vi "BK Precision 178XB Setup Output.vi"() -> ()   [LabVIEW 2019]
doc: "This example VI demonstrates the basic configuration of the power supply. It can be used to configure the voltage and current limit for output, and enables the output once configured."
uses:
  BK Precision 178XB Series.lvlib
panel:
  in  "stop":bool
  in  "Output Voltage (0)":dbl min=0.0 max=18.0 format="%#.2f"
  in  "Current Limit (0)":dbl min=0.0 max=6.0 format="%#.2g"
  in  "Maximum Output Voltage (18)":dbl=8.0 min=0.0 max=72.0 format="%#.2f"
  in  "VISA resource name":refnum<visa-resource-name>
  # "Instructions:  Set the maximum output voltage desired for overvoltage protection.  Then configure the output voltage and the current limit.  To end, press the Stop button."
  # "(c) 2009 B&K PRECISION CORPORATION.  ALL RIGHTS RESERVED."
  # "V"
  # "A"
  # "V"
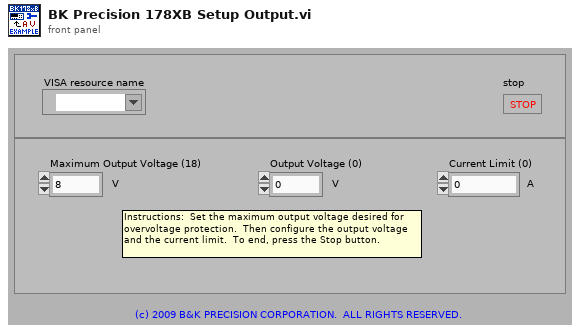
[diagram p1: front panel]
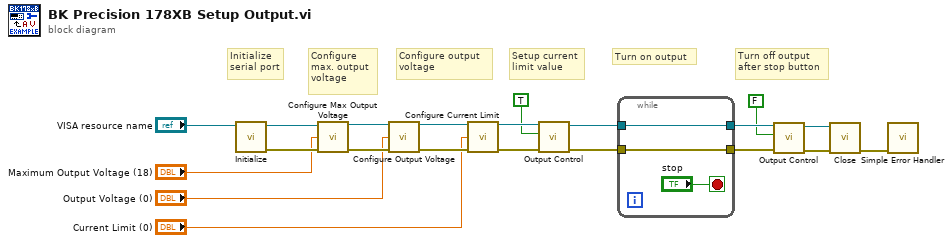
[diagram p0: block diagram]
diagram:
  # "Turn off output\nafter stop button"
  # "Turn on output"
  # "Setup current\nlimit value"
  # "Configure output\nvoltage"
  # "Configure\nmax. output\nvoltage"
  # "Initialize\nserial port"
  n1 = call "Initialize.vi"("VISA resource name"="VISA resource name") -> ("error out"=w19:errorcluster, "VISA resource name out"=w20:refnum<visa-resource-name>)  [unwired: 9 in]
  n2 = call "Configure Max Output Voltage.vi"("VISA resource name"=w20, "Maximum Output Voltage (18)"="Maximum Output Voltage (18)", "error in (no error)"=w19) -> ("VISA resource name out"=w18:refnum<visa-resource-name>, "error out"=w15:errorcluster)  [unwired: 11 in]
  n3 = call "Configure Output Voltage.vi"("VISA resource name"=w18, "Output Voltage (0)"="Output Voltage (0)", "error in (no error)"=w15) -> ("VISA resource name out"=w17:refnum<visa-resource-name>, "error out"=w16:errorcluster)  [unwired: 11 in]
  n4 = call "Configure Current Limit.vi"("VISA resource name"=w17, "Current Limit (0)"="Current Limit (0)", "error in (no error)"=w16) -> ("VISA resource name out"=w14:refnum<visa-resource-name>, "error out"=w13:errorcluster)  [unwired: 11 in]
  n5 = call "Output Control.vi"("error in (no error)"=w13, "Enable Output Terminals (F: Off)"=TRUE, "VISA resource name"=w14) -> ("error out"=w11:errorcluster, "VISA resource name out"=w12:refnum<visa-resource-name>)  [unwired: 7 in]
  n6 = while {
    tunnel: w12 -> [w24]
    tunnel: w11 -> [w23]
    tunnel: [w24] -> w5
    tunnel: [w23] -> w4
    stop <- "stop" stop-if-true
  }
  n7 = call "Output Control.vi"("error in (no error)"=w4, "Enable Output Terminals (F: Off)"=FALSE, "VISA resource name"=w5) -> ("error out"=w2:errorcluster, "VISA resource name out"=w3:refnum<visa-resource-name>)  [unwired: 7 in]
  n8 = call "Close.vi"("error in (no error)"=w2, "VISA resource name"=w3) -> ("error out"=w10:errorcluster)  [unwired: 9 in]
  n9 = call <vilib>:"Simple Error Handler.vi"("error in (no error)"=w10) -> ()  [unwired: 4 in, 5 out]
